vi "Advance past Number.vi"(7 "JSON":string, 9 "Offset (0)":i32, 11 "Parser State in":T1=enum."Number/Other") -> (1 "Offset past match":i32, 3 "Parser State":T1, 6 "Value start out":i32)   [LabVIEW 2015, in "JSONtext.lvlib"]
uses:
  JSONtext.lvlib
  Parsing State.ctl
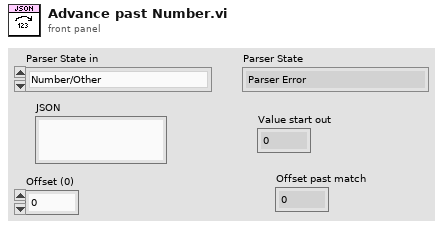
[diagram p1: front panel]
types:
  T1 = typedef "JSONtext.lvlib/Parsing State.ctl" = enum16{"Parser Error", "Object", "Array", "String", "Number/Other", "Leading Whitespace", "Object end", "Array end", "Value end"}
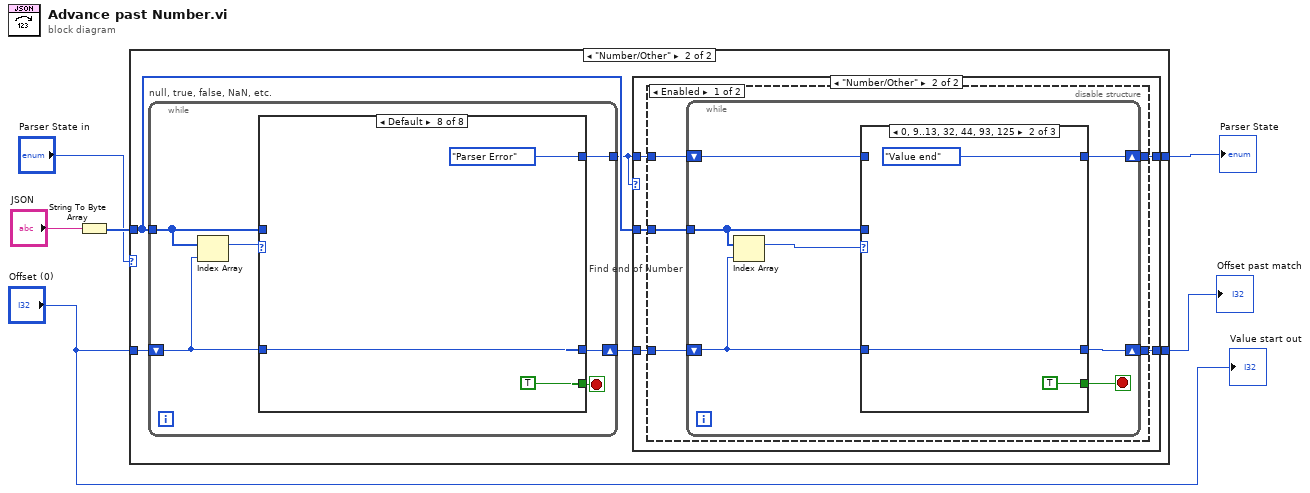
[diagram p0: block diagram]
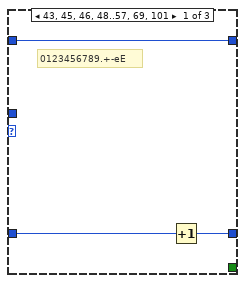
[diagram p4: hidden frame]
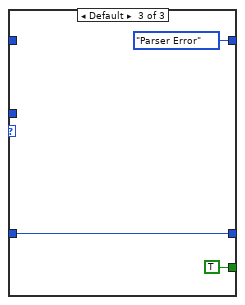
[diagram p5: hidden frame]
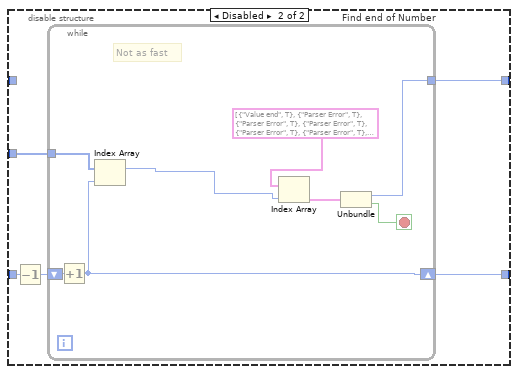
[diagram p6: hidden frame]
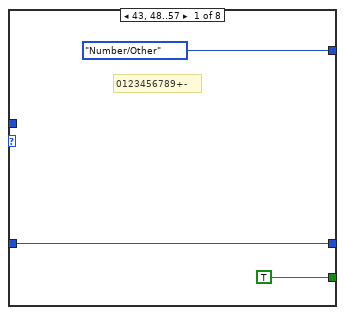
[diagram p7: hidden frame]
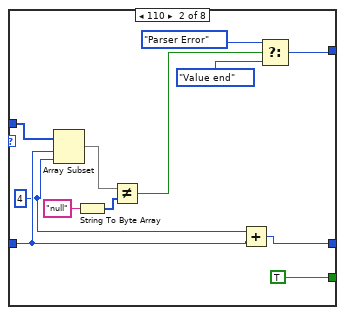
[diagram p8: hidden frame]
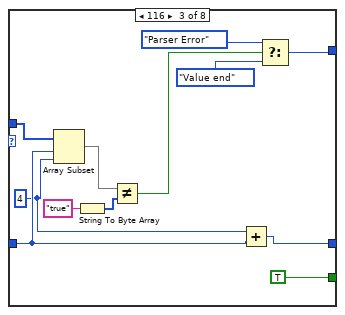
[diagram p9: hidden frame]
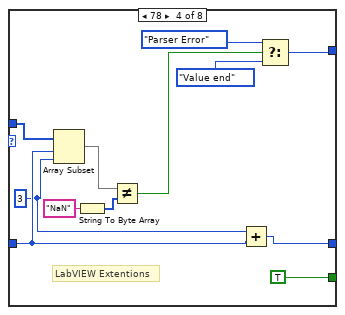
[diagram p10: hidden frame]
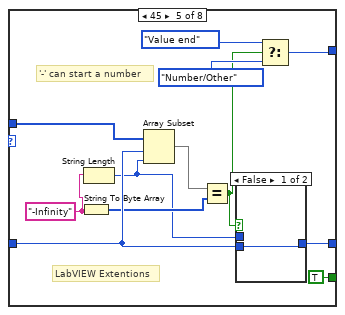
[diagram p11: hidden frame]
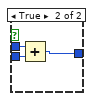
[diagram p12: hidden frame]
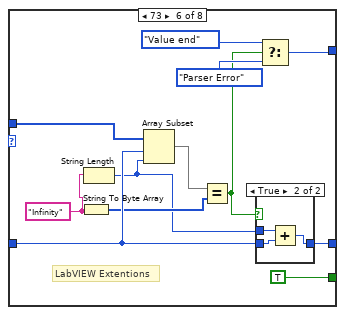
[diagram p13: hidden frame]
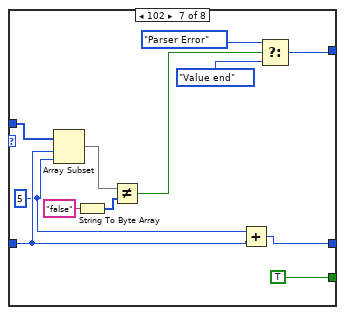
[diagram p15: hidden frame]
diagram:
  n1 = String To Byte Array(string="JSON") -> (unsigned byte array=w2:u8[])
  n2 = case shown="\"Number/Other\"" "Parser State in" {
    tunnel: [_ w13] -> w6
    tunnel: [w7 w12] -> w5
    tunnel: w2 -> [_ w10]
    tunnel: "Offset (0)" -> [w7 w8]
    frame "Parser Error", Default {
    }
    frame "Number/Other" {
      n3 = while "null, true, false, NaN, etc." {
        tunnel: w10 -> [w59]
        shift-right: [w55] -> w11
        shift-left: w8 -> [w56]
        tunnel: [w58] -> w9
        stop <- w57 stop-if-true
        n4 = Index Array(array=w59, index=w56) -> (element=w60:u8)
        n5 = case shown="Default" w60 {
          tunnel: w59 -> [_ w74 w86 w98 w111 w127 w142 _]
          tunnel: [Parsing_State."Number/Other" w71 w83 w95 w109 w125 w139 Parsing_State."Parser Error"] -> w58
          tunnel: [TRUE TRUE TRUE TRUE TRUE TRUE TRUE TRUE] -> w57
          tunnel: w56 -> [w61 w66 w78 w90 w105 w121 w134 w146]
          tunnel: [w61 w64 w76 w88 w104 w120 w132 w146] -> w55
          frame 43, 48..57 {
            # "0123456789+-"
          }
          frame 110 {
            w65 = 4 ("length")
            n6 = Array Subset(array=w74, index=w66, length=w65) -> (w72:u8[])
            n7 = String To Byte Array(string="null") -> (unsigned byte array=w73:u8[])
            n8 = Not Equal?(x=w72, y=w73) -> (x != y?=w68:bool)
            n9 = Add(x=w65, y=w66) -> (x+y=w64:i32)
            n10 = Select(t=Parsing_State."Parser Error", s=w68, f=Parsing_State."Value end") -> (s? t:f=w71:T1)
          }
          frame 116 {
            w77 = 4 ("length")
            n11 = Array Subset(array=w86, index=w78, length=w77) -> (w84:u8[])
            n12 = String To Byte Array(string="true") -> (unsigned byte array=w85:u8[])
            n13 = Not Equal?(x=w84, y=w85) -> (x != y?=w80:bool)
            n14 = Add(x=w77, y=w78) -> (x+y=w76:i32)
            n15 = Select(t=Parsing_State."Parser Error", s=w80, f=Parsing_State."Value end") -> (s? t:f=w83:T1)
          }
          frame 78 {
            w89 = 3 ("length")
            # "LabVIEW Extentions"
            n16 = Array Subset(array=w98, index=w90, length=w89) -> (w96:u8[])
            n17 = String To Byte Array(string="NaN") -> (unsigned byte array=w97:u8[])
            n18 = Not Equal?(x=w96, y=w97) -> (x != y?=w92:bool)
            n19 = Add(x=w89, y=w90) -> (x+y=w88:i32)
            n20 = Select(t=Parsing_State."Parser Error", s=w92, f=Parsing_State."Value end") -> (s? t:f=w95:T1)
          }
          frame 45 {
            w102 = "-Infinity"
            # "'-' can start a number"
            # "LabVIEW Extentions"
            n21 = String To Byte Array(string=w102) -> (unsigned byte array=w103:u8[])
            n22 = String Length(string=w102) -> (length=w101:i32)
            n23 = Array Subset(array=w111, index=w105, length=w101) -> (w110:u8[])
            n24 = Equal?(x=w110, y=w103) -> (x = y?=w100:bool)
            n25 = case shown="False" w100 {
              tunnel: w105 -> [w112 w115]
              tunnel: [w112 w114] -> w104
              tunnel: w101 -> [_ w113]
              frame False {
              }
              frame True {
                n26 = Add(x=w113, y=w115) -> (x+y=w114:i32)
              }
            }
            n27 = Select(t=Parsing_State."Value end", s=w100, f=Parsing_State."Number/Other") -> (s? t:f=w109:T1)
          }
          frame 73 {
            w118 = "Infinity"
            # "LabVIEW Extentions"
            n28 = String To Byte Array(string=w118) -> (unsigned byte array=w119:u8[])
            n29 = String Length(string=w118) -> (length=w117:i32)
            n30 = Array Subset(array=w127, index=w121, length=w117) -> (w126:u8[])
            n31 = Equal?(x=w126, y=w119) -> (x = y?=w116:bool)
            n32 = case shown="True" w116 {
              tunnel: w121 -> [w128 w131]
              tunnel: [w128 w130] -> w120
              tunnel: w117 -> [_ w129]
              frame False {
              }
              frame True {
                n33 = Add(x=w129, y=w131) -> (x+y=w130:i32)
              }
            }
            n34 = Select(t=Parsing_State."Value end", s=w116, f=Parsing_State."Parser Error") -> (s? t:f=w125:T1)
          }
          frame 102 {
            w133 = 5 ("length")
            n35 = Array Subset(array=w142, index=w134, length=w133) -> (w140:u8[])
            n36 = String To Byte Array(string="false") -> (unsigned byte array=w141:u8[])
            n37 = Not Equal?(x=w140, y=w141) -> (x != y?=w136:bool)
            n38 = Add(x=w133, y=w134) -> (x+y=w132:i32)
            n39 = Select(t=Parsing_State."Parser Error", s=w136, f=Parsing_State."Value end") -> (s? t:f=w139:T1)
          }
          frame Default {
          }
        }
      }
      n40 = case shown="\"Number/Other\"" w9 {
        tunnel: [w14 w20] -> w13
        tunnel: [w15 w19] -> w12
        tunnel: w11 -> [w15 w16]
        tunnel: w9 -> [w14 w18]
        tunnel: w10 -> [_ w17]
        frame "Parser Error", Default {
        }
        frame "Number/Other" {
          n41 = disable-structure shown="Enabled" {
            disable-tunnel: [w25 w46] -> w20
            disable-tunnel: [w24 w45] -> w19
            disable-tunnel: w18 -> [w23 _]
            disable-tunnel: w17 -> [w22 w44]
            disable-tunnel: w16 -> [w21 w43]
            frame Enabled {
              n42 = while "Find end of Number" {
                tunnel: w22 -> [w32]
                shift-right: [w28] -> w24
                shift-left: w21 -> [w26]
                shift-right: [w30] -> w25
                shift-left: w23 -> [w31]
                stop <- w29 stop-if-true
                n43 = Index Array(array=w32, index=w26) -> (element=w27:u8)
                n44 = case shown="0, 9..13, 32, 44, 93, 125" w27 {
                  tunnel: w32 -> [_ _ _]
                  tunnel: w31 -> [w35 _ _]
                  tunnel: [w35 Parsing_State."Value end" Parsing_State."Parser Error"] -> w30
                  tunnel: [_ TRUE TRUE] -> w29
                  tunnel: w26 -> [w34 w36 w41]
                  tunnel: [w33 w36 w41] -> w28
                  frame 43, 45, 46, 48..57, 69, 101 {
                    # "0123456789.+-eE"
                    n45 = Increment(x=w34) -> (x+1=w33:i32)
                  }
                  frame 0, 9..13, 32, 44, 93, 125 {
                  }
                  frame Default {
                  }
                }
              }
            }
            frame Disabled {
              n46 = Decrement(x=w43) -> (x-1=w42:i32)
              n47 = while "Find end of Number" {
                tunnel: w44 -> [w54]
                shift-right: [w47] -> w45
                shift-left: w42 -> [w53]
                tunnel: [w48] -> w46
                stop <- w49 stop-if-true
                # "Not as fast"
                n48 = Increment(x=w53) -> (x+1=w47:i32)
                n49 = Index Array(array=w54, index=w47) -> (element=w50:u8)
                n50 = Index Array(array=cluster{T1, bool}[] [{enum."Value end", TRUE}, {enum."Parser Error", TRUE}, {enum."Parser Error", TRUE}, {enum."Parser Error", TRUE}, {enum."Parser Error", TRUE}, {enum."Parser Error", TRUE}, {enum."Parser Error", TRUE}, {enum."Parser Error", TRUE}, {enum."Parser Error", TRUE}, {enum."Value end", TRUE}, {enum."Value end", TRUE}, {enum."Value end", TRUE}, {enum."Value end", TRUE}, {enum."Value end", TRUE}, {enum."Parser Error", TRUE}, {enum."Parser Error", TRUE}, {enum."Parser Error", TRUE}, {enum."Parser Error", TRUE}, {enum."Parser Error", TRUE}, {enum."Parser Error", TRUE}, {enum."Parser Error", TRUE}, {enum."Parser Error", TRUE}, {enum."Parser Error", TRUE}, {enum."Parser Error", TRUE}, {enum."Parser Error", TRUE}, {enum."Parser Error", TRUE}, {enum."Parser Error", TRUE}, {enum."Parser Error", TRUE}, {enum."Parser Error", TRUE}, {enum."Parser Error", TRUE}, {enum."Parser Error", TRUE}, {enum."Parser Error", TRUE}, {enum."Value end", TRUE}, {enum."Parser Error", TRUE}, {enum."Parser Error", TRUE}, {enum."Parser Error", TRUE}, {enum."Parser Error", TRUE}, {enum."Parser Error", TRUE}, {enum."Parser Error", TRUE}, {enum."Parser Error", TRUE}, {enum."Parser Error", TRUE}, {enum."Parser Error", TRUE}, {enum."Parser Error", TRUE}, {enum."Number/Other", FALSE}, {enum."Value end", TRUE}, {enum."Number/Other", FALSE}, {enum."Number/Other", FALSE}, {enum."Parser Error", TRUE}, {enum."Number/Other", FALSE}, {enum."Number/Other", FALSE}, {enum."Number/Other", FALSE}, {enum."Number/Other", FALSE}, {enum."Number/Other", FALSE}, {enum."Number/Other", FALSE}, {enum."Number/Other", FALSE}, {enum."Number/Other", FALSE}, {enum."Number/Other", FALSE}, {enum."Number/Other", FALSE}, {enum."Parser Error", TRUE}, {enum."Parser Error", TRUE}, {enum."Parser Error", TRUE}, {enum."Parser Error", TRUE}, {enum."Parser Error", TRUE}, {enum."Parser Error", TRUE}, {enum."Parser Error", TRUE}, {enum."Parser Error", TRUE}, {enum."Parser Error", TRUE}, {enum."Parser Error", TRUE}, {enum."Parser Error", TRUE}, {enum."Number/Other", FALSE}, {enum."Parser Error", TRUE}, {enum."Parser Error", TRUE}, {enum."Parser Error", TRUE}, {enum."Parser Error", TRUE}, {enum."Parser Error", TRUE}, {enum."Parser Error", TRUE}, {enum."Parser Error", TRUE}, {enum."Parser Error", TRUE}, {enum."Parser Error", TRUE}, {enum."Parser Error", TRUE}, {enum."Parser Error", TRUE}, {enum."Parser Error", TRUE}, {enum."Parser Error", TRUE}, {enum."Parser Error", TRUE}, {enum."Parser Error", TRUE}, {enum."Parser Error", TRUE}, {enum."Parser Error", TRUE}, {enum."Parser Error", TRUE}, {enum."Parser Error", TRUE}, {enum."Parser Error", TRUE}, {enum."Parser Error", TRUE}, {enum."Parser Error", TRUE}, {enum."Parser Error", TRUE}, {enum."Value end", TRUE}, {enum."Parser Error", TRUE}, {enum."Parser Error", TRUE}, {enum."Parser Error", TRUE}, {enum."Parser Error", TRUE}, {enum."Parser Error", TRUE}, {enum."Parser Error", TRUE}, {enum."Parser Error", TRUE}, {enum."Number/Other", FALSE}, {enum."Parser Error", TRUE}, {enum."Parser Error", TRUE}, {enum."Parser Error", TRUE}, {enum."Parser Error", TRUE}, {enum."Parser Error", TRUE}, {enum."Parser Error", TRUE}, {enum."Parser Error", TRUE}, {enum."Parser Error", TRUE}, {enum."Parser Error", TRUE}, {enum."Parser Error", TRUE}, {enum."Parser Error", TRUE}, {enum."Parser Error", TRUE}, {enum."Parser Error", TRUE}, {enum."Parser Error", TRUE}, {enum."Parser Error", TRUE}, {enum."Parser Error", TRUE}, {enum."Parser Error", TRUE}, {enum."Parser Error", TRUE}, {enum."Parser Error", TRUE}, {enum."Parser Error", TRUE}, {enum."Parser Error", TRUE}, {enum."Parser Error", TRUE}, {enum."Parser Error", TRUE}, {enum."Value end", TRUE}] ("Array"), index=w50) -> (element=w51:cluster{T1, bool})
                n51 = Unbundle(w51) -> (w48:T1, w49:bool)
              }
            }
          }
        }
      }
    }
  }
  "Parser State" <- w6
  "Offset past match" <- w5
  "Value start out" <- "Offset (0)"
